vi "AssertImage.vi"(11 "Image Src Reference In":T1) -> (3 "Image Reference Out":T1)   [LabVIEW 2020, in "OpenLvVision_OpenCv.lvlib"]
uses:
  OpenLvVision_OpenCv.lvlib
  <vilib>/OpenLvVision/OpenLvVision_Image/Management/TypeDef/OLV Image.ctl
  <vilib>/OpenLvVision/OpenLvVision_Image/Management/OLV Management.lvlib
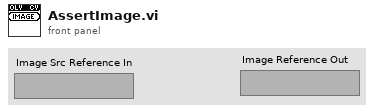
[diagram p1: front panel]
types:
  T1 = typedef "OLV OpenLvVision_Image.lvlib/OLV Management.lvlib/OLV Image.ctl" = refnum<image>
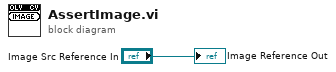
[diagram p0: block diagram]
diagram:
  "Image Reference Out" <- "Image Src Reference In"
